vi "errmsg.vi"(8 "error in (no error)":errorcluster, 11 "para0":u64) -> (0 "error out":errorcluster, 2 "function return":string, 3 "para0 out":u64)   [LabVIEW 2020, in "sqlite3.lvlib"]
uses:
  sqlite3.lvlib
  bin/sqlite3_64.dll
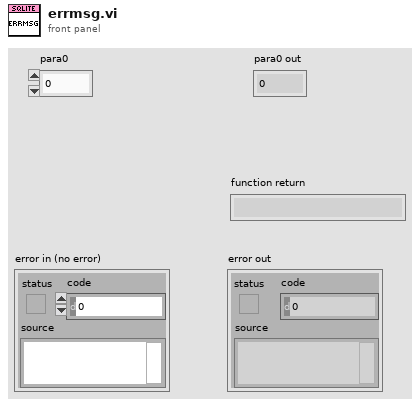
[diagram p1: front panel]
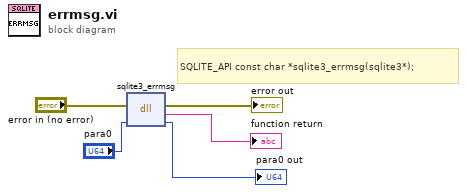
[diagram p0: block diagram]
diagram:
  # "SQLITE_API const char *sqlite3_errmsg(sqlite3*);"
  n1 = dll-call lib="C:/Users/Fred.Guo/Desktop/Database-configuration/externals/sqlite3/Source/bin/sqlite3_*.*" fn="sqlite3_errmsg"(error in="error in (no error)", "para0"="para0") -> (error out=→"error out":errorcluster, "return type"=→"function return":string, "para0"=→"para0 out":u64)  [unwired: 2 in, 1 out]
